vi "Process Lidar Data (Library Call).vi"(6 "Pose Delta":cluster{"X":dbl, "Y":dbl, "R":dbl}, 9 "Direction":dbl[](array[numeric]), 10 "Magnitude":dbl[](array[numeric]), 11 "Library Path":path) -> (2 "Y":dbl[](array[numeric]), 3 "X":dbl[](array[numeric]))   [LabVIEW 2018]
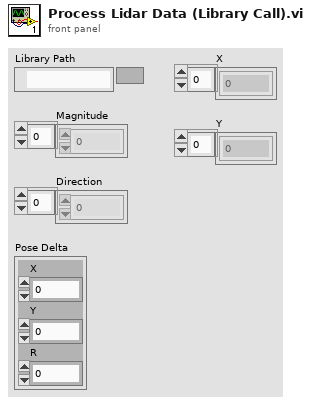
[diagram p1: front panel]
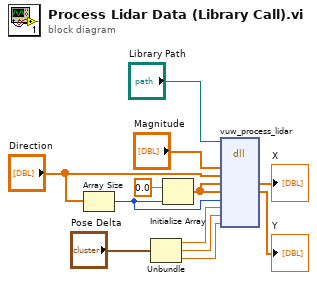
[diagram p0: block diagram]
diagram:
  n1 = Array Size(array="Direction") -> (size(s)=w6:i32)
  n2 = Unbundle("Pose Delta") -> ("X"=w2:dbl, "Y"=w1:dbl, "R"=w9:dbl)
  n3 = Initialize Array(0.0 ("element"), w6) -> (w5:dbl[])
  n4 = dll-call lib="home/admin/lib/libslam.so" fn="vuw_process_lidar"(path in="Library Path", "magnitude"="Magnitude", "theta"="Direction", "out_x"=w5, "out_y"=w5, "nb_points"=w6, "d_x"=w2, "d_y"=w1, "d_theta"=w9) -> ("out_x"=→"X":sgl[], "out_y"=→"Y":sgl[])  [unwired: 9 in, 2 out]
